vi "rqcAlice Create ServiceNET.vi"(8 "error in":errorcluster, 10 "port":u16) -> (0 "error out":errorcluster, 3 "rqcAlice ServiceNET control":T1)   [LabVIEW 2018]
uses:
  Custom Controls/rqcAlice ServiceNET control.ctl
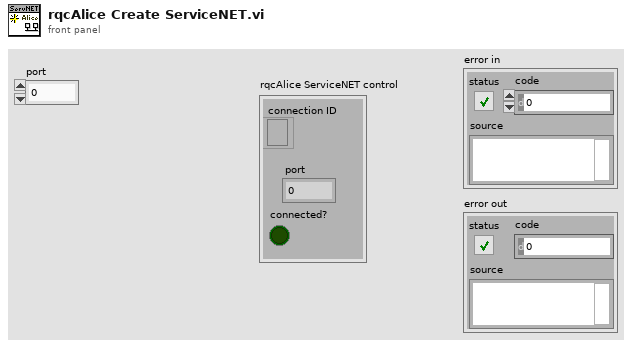
[diagram p1: front panel]
types:
  T1 = typedef "rqcAlice ServiceNET control.ctl" = cluster{"connection ID":refnum<k5>, "port":u16, "connected?":bool}
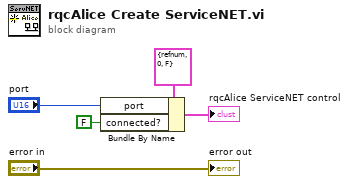
[diagram p0: block diagram]
diagram:
  n1 = Bundle By Name(cluster=T1 {"connection ID"=refnum, "port"=0, "connected?"=FALSE} ("rqcAlice ServiceNET control"), "port"="port", "connected?"=FALSE) -> (→"rqcAlice ServiceNET control":T1)
  "error out" <- "error in"
